vi "PH_Beckhoff_PP_PU.declare digital InputTags.vi"(2 "Instance Name":string="N/A", 4 "PU Type":T2) -> (0 "Digital Inputs":T3, 1 "Description":string)   [LabVIEW 2014, in "PH_Beckhoff_PP_PU.lvlib"]
uses:
  PH_Beckhoff_PP_PU.lvlib
  PH_Beckhoff/PH_Beckhoff.Digital Inputs.ctl
  PH_Beckhoff_PP_PU.PU Rack Type.ctl
  PH_PP_Common/PH_PP_Common.PSU Tags.ctl
  PH_Beckhoff_PP_PU.Igni Tags.ctl
  PH_Beckhoff_PP_PU.RR Tags.ctl
  PH_PP_Common/PH_PP_Common.Trigger Tags.ctl
  PH_PP_Common/PH_PP_Common.PUs.ctl
  PH_PP_Common/PH_PP_Common.PSU Type.ctl
  PH_Beckhoff/PH_Beckhoff.lvlib
  PH_PP_Common/PH_PP_Common.lvlib
panel:
  in  "Digital Input Value":T1
  out "Right Size?":bool
  # "Let this VI run to check the size!"
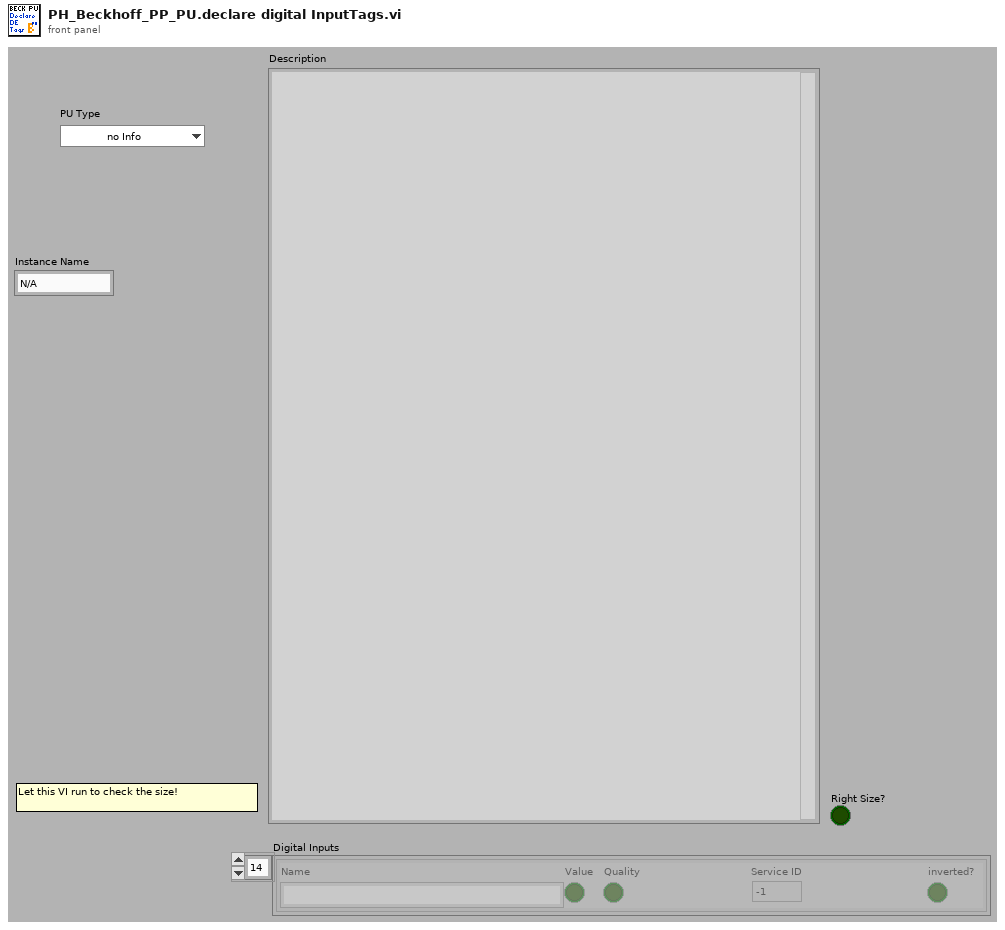
[diagram p1: front panel]
types:
  T1 = cluster{"Name":string, "Value":bool, "Quality":bool, "Service ID":i32, "inverted?":bool}
  T2 = typedef "PH_Beckhoff_PP_PU.lvlib/PH_Beckhoff_PP_PU.PU Rack Type.ctl" = enum16{"no Info", "PA 19mm", "PA 45mm", "MA PU 1 and 2", "MA PU 3 and 4", "MA PU 5 and 6", "MA FR and PILC"}
  T3 = typedef "PH_Beckhoff.lvlib/PH_Beckhoff.Digital Inputs.ctl" = cluster{"Name":string, "Value":bool, "Quality":bool, "Service ID":i32, "inverted?":bool}[]
  T4 = typedef "PH_PP_Common.lvlib/PH_PP_Common.PUs.ctl" = enum16{"no Info", "PA-19mm-1", "PA-19mm-2", "PA-45mm-PILC", "PA-45mm-MAIN", "MA-PU-1", "MA-PU-2", "MA-PU-3", "MA-PU-4", "MA-PU-5", "MA-PU-6", "MA-FR", "MA-PILC", "PA-45mm-DP"}
  T5 = typedef "PH_Beckhoff_PP_PU.lvlib/PH_Beckhoff_PP_PU.Igni Tags.ctl" = enum16{"heating-on", "water-on", "Device-on", "Status"}
  T6 = typedef "PH_PP_Common.lvlib/PH_PP_Common.PSU Tags.ctl" = enum16{"voltage-indicator", "peak-detect", "current", "voltage", "inihibit-indicator", "end-of-charge", "HV-on-indicator", "overtemperature", "interlock-indicator", "load-fault", "sum-fault", "HV-off-indicator", "DC-ok", "inhibit", "HV-on", "interlock", "reset", "Status", "Limits"}
  T7 = typedef "PH_PP_Common.lvlib/PH_PP_Common.Trigger Tags.ctl" = enum16{"triggered", "fired", "Status", "Last Shot"}
  T8 = typedef "PH_Beckhoff_PP_PU.lvlib/PH_Beckhoff_PP_PU.RR Tags.ctl" = enum16{"open", "closed", "close", "Status"}
  T9 = typedef "PH_PP_Common.lvlib/PH_PP_Common.PSU Type.ctl" = enum16{"none", "Maxwell Standard", "DEL", "Maxwell ALE", "Continuum 601k"}
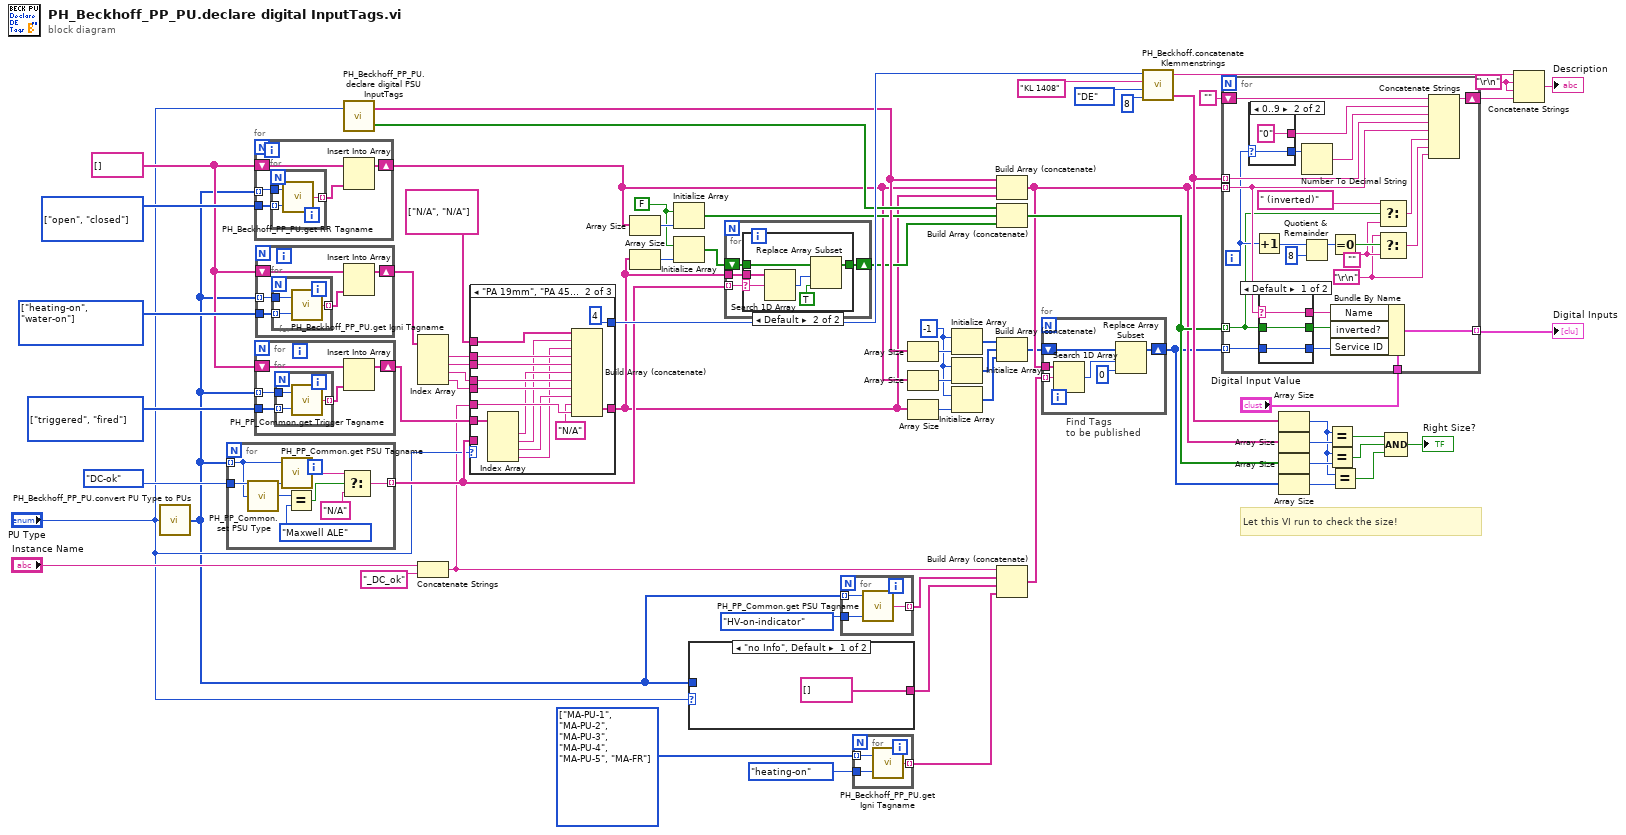
[diagram p0: block diagram]
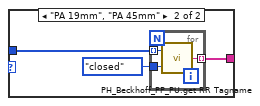
[diagram p2: hidden frame]
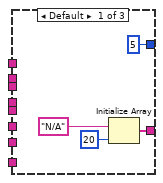
[diagram p4: hidden frame]
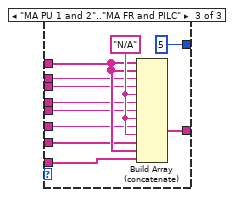
[diagram p5: hidden frame]
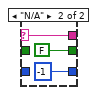
[diagram p6: hidden frame]
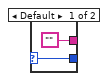
[diagram p7: hidden frame]
diagram:
  w1 = T4[] [enum."MA-PU-1", enum."MA-PU-2", enum."MA-PU-3", enum."MA-PU-4", enum."MA-PU-5", enum."MA-FR"] items=["no Info", "PA-19mm-1", "PA-19mm-2", "PA-45mm-PILC", "PA-45mm-MAIN", "MA-PU-1", "MA-PU-2", "MA-PU-3", "MA-PU-4", "MA-PU-5", "MA-PU-6", "MA-FR", "MA-PILC", "PA-45mm-DP"] ("PUs")
  w27 = T7[] [enum."triggered", enum."fired"] items=["triggered", "fired", "Status", "Last Shot"]
  w21 = FALSE
  w32 = T8[] [enum."open", enum."closed"] items=["open", "closed", "close", "Status"]
  w37 = T5[] [enum."heating-on", enum."water-on"] items=["heating-on", "water-on", "Device-on", "Status"]
  w20 = -1 ("Service ID")
  w26 = string[] []
  w64 = "\r\n"
  # "Let this VI run to check the size!"
  n1 = call "PH_Beckhoff_PP_PU.convert PU Type to PUs.vi"("PU Type"="PU Type") -> ("PUs"=w4:T4[])
  n2 = for "PSU" {
    tunnel: [w71] -> w19 mode=indexing
    tunnel: w4 -> [w68] mode=indexing
    tunnel: PH_PP_Common.PSU_Tags."DC-ok" ("PSU Tag") -> [w70]
    n3 = call "PH_PP_Common.set PSU Type.vi"("PU"=w68) -> ("PSU Type"=w67:T9)
    n4 = call "PH_PP_Common.get PSU Tagname.vi"("PSU Tag"=w70, "PU"=w68) -> ("PSU Tagname"=w69:string)  [unwired: 1 in]
    n5 = Equal?(x=w67, y=PH_PP_Common.PSU_Type."Maxwell ALE") -> (x = y?=w73:bool)
    n6 = Select(t=w69, s=w73, f="N/A") -> (s? t:f=w71:string)
  }
  n7 = for "Ross Relais" {
    shift-right: [w79] -> w18
    shift-left: w26 -> [w78]
    tunnel: w4 -> [w77] mode=indexing
    tunnel: w32 -> [w76]
    n8 = for {
      tunnel: w77 -> [w82]
      tunnel: w76 -> [w81] mode=indexing
      tunnel: [w80] -> w75 mode=indexing
      n9 = call "PH_Beckhoff_PP_PU.get RR Tagname.vi"("Ross Relais Tag"=w81, "PU"=w82) -> ("RR Tagname"=w80:string)
    }
    n10 = Insert Into Array(array=w78, new element=w75) -> (w79:string[])  [unwired: 1 in]
  }
  n11 = for "Trigger" {
    shift-right: [w87] -> w25
    shift-left: w26 -> [w85]
    tunnel: w4 -> [w84] mode=indexing
    tunnel: w27 -> [w83]
    n12 = for {
      tunnel: [w90] -> w86 mode=indexing
      tunnel: w84 -> [w89]
      tunnel: w83 -> [w88] mode=indexing
      n13 = call "PH_PP_Common.get Trigger Tagname.vi"("Trigger Tag"=w88, "PU"=w89) -> ("Trigger Tagname"=w90:string)
    }
    n14 = Insert Into Array(array=w85, new element=w86) -> (w87:string[])  [unwired: 1 in]
  }
  n15 = for "Igni" {
    shift-right: [w95] -> w24
    shift-left: w26 -> [w93]
    tunnel: w4 -> [w92] mode=indexing
    tunnel: w37 -> [w91]
    n16 = for {
      tunnel: [w98] -> w94 mode=indexing
      tunnel: w92 -> [w97]
      tunnel: w91 -> [w96] mode=indexing
      n17 = call "PH_Beckhoff_PP_PU.get Igni Tagname.vi"("Igni Tag"=w96, "PU"=w97) -> ("Igni Tagname"=w98:string)
    }
    n18 = Insert Into Array(array=w93, new element=w94) -> (w95:string[])  [unwired: 1 in]
  }
  n19 = call "PH_Beckhoff_PP_PU.declare digital PSU InputTags.vi"("PUs"="PU Type") -> ("inverted"=w42:bool[], "Tagnames"=w40:string[])  [unwired: 1 in]
  n20 = Index Array(array=w24) -> (element #1=w36:string, element #2=w35:string, element #3=w34:string, element #4=w33:string)  [unwired: 4 in]
  n21 = Concatenate Strings("Instance Name", "_DC_ok" ("string")) -> (w5:string)
  n22 = case "PU" shown="\"PA 19mm\", \"PA 45mm\"" "PU Type" {
    tunnel: [5 ("Quantity") 4 ("Quantity") 5 ("Quantity")] -> w46
    tunnel: string[] ["N/A", "N/A"] -> [_ w114 w124]
    tunnel: [w99 w108 w126] -> w15
    tunnel: w5 -> [_ w115 w123]
    tunnel: w19 -> [_ _ w122]
    tunnel: w36 -> [_ w113 w121]
    tunnel: w35 -> [_ w112 w120]
    tunnel: w34 -> [_ w111 w119]
    tunnel: w33 -> [_ w110 w118]
    tunnel: w25 -> [_ w107 w117]
    frame Default {
      n23 = Initialize Array("N/A", 20 ("dimension size")) -> (w99:string[])
    }
    frame "PA 19mm", "PA 45mm" {
      n24 = Index Array(array=w107) -> (element #1=w106:string, element #2=w105:string, element #3=w104:string, element #4=w103:string)  [unwired: 4 in]
      n25 = Build Array (concatenate)(w114, w105, w103, w113, w112, w106, w111, w110, w104, "N/A", w115) -> (w108:string[])
    }
    frame "MA PU 1 and 2".."MA FR and PILC" {
      w125 = "N/A"
      n26 = Build Array (concatenate)(w124, w124, w121, w120, w125, w119, w118, w125, w123, w125, w117, w124, w122) -> (w126:string[])
    }
  }
  n27 = Array Size(array=w18) -> (size(s)=w29:i32)
  n28 = Array Size(array=w15) -> (size(s)=w23:i32)
  n29 = Initialize Array(w21, w29) -> (w28:bool[])
  n30 = Initialize Array(w21, w23) -> (w17:bool[])
  n31 = case shown="\"no Info\", Default" "PU Type" {
    tunnel: [string[] [] w131] -> w9
    tunnel: w4 -> [_ w129]
    frame "no Info", Default {
    }
    frame "PA 19mm", "PA 45mm" {
      n32 = for {
        tunnel: w129 -> [w134] mode=indexing
        tunnel: PH_Beckhoff_PP_PU.RR_Tags."closed" ("Ross Relais Tag") -> [w133]
        tunnel: [w132] -> w131 mode=indexing
        n33 = call "PH_Beckhoff_PP_PU.get RR Tagname.vi"("Ross Relais Tag"=w133, "PU"=w134) -> ("RR Tagname"=w132:string)
      }
    }
  }
  n34 = for {
    tunnel: w19 -> [w137] mode=indexing
    tunnel: w15 -> [w138]
    shift-right: [w135] -> w16
    shift-left: w17 -> [w136]
    n35 = case shown="Default" w137 {
      selector: w137 -> [_ w144]
      tunnel: w138 -> [_ w145]
      tunnel: w136 -> [w139 w143]
      tunnel: [w139 w141] -> w135
      frame "N/A" {
      }
      frame Default {
        n36 = Search 1D Array(1D array=w145, element=w144) -> (index of element=w142:i32)  [unwired: 1 in]
        n37 = Replace Array Subset(array=w143, new element=TRUE ("new element/subarray"), index=w142) -> (w141:bool[])
      }
    }
  }
  n38 = for "PSU" {
    tunnel: w4 -> [w148] mode=indexing
    tunnel: PH_PP_Common.PSU_Tags."HV-on-indicator" ("PSU Tag") -> [w147]
    tunnel: [w146] -> w7 mode=indexing
    n39 = call "PH_PP_Common.get PSU Tagname.vi"("PSU Tag"=w147, "PU"=w148) -> ("PSU Tagname"=w146:string)  [unwired: 1 in]
  }
  n40 = for {
    tunnel: [w151] -> w2 mode=indexing
    tunnel: w1 -> [w150] mode=indexing
    tunnel: PH_Beckhoff_PP_PU.Igni_Tags."heating-on" ("Igni Tag") -> [w149]
    n41 = call "PH_Beckhoff_PP_PU.get Igni Tagname.vi"("Igni Tag"=w149, "PU"=w150) -> ("Igni Tagname"=w151:string)
  }
  n42 = Array Size(array=w40) -> (size(s)=w39:i32)
  n43 = Array Size(array=w18) -> (size(s)=w31:i32)
  n44 = Array Size(array=w15) -> (size(s)=w22:i32)
  n45 = Initialize Array(w20, w39) -> (w38:i32[])
  n46 = Initialize Array(w20, w31) -> (w30:i32[])
  n47 = Initialize Array(w20, w22) -> (w14:i32[])
  n48 = Build Array (concatenate)(w40, w18, w15) -> (w13:string[])
  n49 = Build Array (concatenate)(w42, w28, w16) -> (w50:bool[])
  n50 = Build Array (concatenate)(w38, w30, w14) -> (w12:i32[])
  n51 = Build Array (concatenate)(w5, w7, w9, w2) -> (w10:string[])
  n52 = for "Find Tags \nto be published" {
    tunnel: w10 -> [w155] mode=indexing
    tunnel: w13 -> [w154]
    shift-right: [w152] -> w11
    shift-left: w12 -> [w153]
    n53 = Search 1D Array(1D array=w154, element=w155) -> (index of element=w157:i32)  [unwired: 1 in]
    n54 = Replace Array Subset(array=w153, new element=0 ("new element/subarray"), index=w157) -> (w152:i32[])
  }
  n55 = call "PH_Beckhoff.concatenate Klemmenstrings.vi"("# of In- or Outputs"=8, "Type"=enum16{"AE", "AA", "DE", "DA", "SE"}."DE", "Klemmenname"="KL 1408", "Quantity"=w46) -> ("concatenated string array"=w59:string[], "\"<Type>: <Quantity> x <Klemmenname>\""=w60:string)  [unwired: 1 out]
  n56 = for {
    tunnel: w13 -> [w174] mode=indexing
    tunnel: w59 -> [w178] mode=indexing
    shift-right: [w160] -> w65
    shift-left: "" -> [w161]
    tunnel: w50 -> [w165] mode=indexing
    tunnel: [w176] -> w52 mode=indexing
    tunnel: "Digital Input Value" -> [w177]
    tunnel: w11 -> [w171] mode=indexing
    i -> [w170]
    w158 = "\r\n"
    w164 = ""
    n57 = case shown="0..9" w170 {
      selector: w170 -> [w188 w191]
      tunnel: [w188 w191] -> w181
      tunnel: ["" "0"] -> w180
      frame Default {
      }
      frame 0..9 {
      }
    }
    n58 = Increment(x=w170) -> (x+1=w169:i32)
    n59 = case shown="Default" w174 {
      selector: w174 -> [w182 w185]
      tunnel: w171 -> [w184 _]
      tunnel: [w184 -1 ("Service ID")] -> w173
      tunnel: w165 -> [w183 _]
      tunnel: [w183 FALSE ("element")] -> w172
      tunnel: [w182 w185] -> w175
      frame Default {
      }
      frame "N/A" {
      }
    }
    n60 = Number To Decimal String(number=w181) -> (decimal integer string=w179:string)  [unwired: 1 in]
    n61 = Quotient & Remainder(x=w169, y=8) -> (x-y*floor(x/y)=w167:i32)  [unwired: 1 out]
    n62 = Equal To 0?(x=w167) -> (x = 0?=w166:bool)
    n63 = Bundle By Name(cluster=w177, "Name"=w175, "inverted?"=w172, "Service ID"=w173) -> (w176:T1)
    n64 = Select(t=" (inverted)" ("string"), s=w165, f=w164) -> (s? t:f=w162:string)
    n65 = Select(t=w158, s=w166, f=w164) -> (s? t:f=w159:string)
    n66 = Concatenate Strings(w161, w180, w179, w178, w174, w162, w159, w158) -> (w160:string)
  }
  "Digital Inputs" <- w52
  n67 = Array Size(array=w59) -> (size(s)=w48:i32)
  n68 = Array Size(array=w13) -> (size(s)=w58:i32)
  n69 = Array Size(array=w50) -> (size(s)=w57:i32)
  n70 = Array Size(array=w11) -> (size(s)=w49:i32)
  n71 = Equal?(x=w48, y=w58) -> (x = y?=w55:bool)
  n72 = Equal?(x=w48, y=w57) -> (x = y?=w54:bool)
  n73 = Equal?(x=w48, y=w49) -> (x = y?=w47:bool)
  n74 = Compound Arithmetic op=AND(w55, w54, w47) -> (→"Right Size?":bool)
  n75 = Concatenate Strings(w60, w64, w64, w65) -> (→"Description":string)
